vi "defaults.vi"(1 "Do this?":bool=TRUE, 2 "Input":i32[][](array[numeric]), 3 "Absolute start time (ms)":dbl format="%.3f") -> (0 "Output":i32[][](array[numeric])=[[0, 0, 0, 0], [0, 0, 0, 0], [0, 0, 0, 0], [0, 0, 0, 0], [0, 0, 0, 0], [0, 0, 0, 0], [0, 0, 0, 0], [0, 0, 0, 0], [0, 0, 0, 0], [0, 0, 0, 0], [0, 0, 0, 0], [0, 0, 0, 0], [0, 0, 0, 0], [0, 0, 0, 0], [0, 0, 0, 0], [0, 0, 0, 0], [0, 0, 0, 0], [0, 0, 0, 0], [0, 0, 0, 0], [0, 0, 0, 0], [0, 0, 0, 0], [0, 0, 0, 0], [0, 0, 0, 1], [0, 0, 0, 1], [0, 0, 0, 1], [0, 0, 0, 1], [0, 0, 0, 1], [0, 0, 0, 1], [0, 0, 0, 1], [0, 0, 0, 1], [0, 0, 0, 1], [0, 0, 0, 1], [0, 0, 0, 1], [0, 0, 1, 0], [0, 0, 2, 0], [0, 0, 3, 0], [0, 0, 4, 0], [0, 0, 5, 1], [0, 0, 6, 1], [0, 0, 7, 1], [0, 0, 8, 0], [0, 0, 9, 1], [0, 0, 10, 0], [0, 0, 11, 0], [0, 0, 12, 0], [0, 0, 13, 0], [0, 0, 14, 1], [0, 0, 15, 1], [0, 1, 0, 1], [0, 1, 1, 1], [0, 1, 2, 0], [0, 1, 3, 0], [0, 1, 4, 0], [0, 1, 5, 1], [0, 1, 6, 0], [0, 1, 7, 0], [0, 1, 8, 0], [0, 1, 9, 0], [0, 1, 10, 1], [0, 1, 11, 0], [0, 1, 12, 1], [0, 1, 13, 0], [0, 1, 14, 0], [0, 1, 15, 0]] caption="time(ms)        port            line               value")   [LabVIEW 2015]
uses:
  globals and logs/board parameters.vi
  globals and logs/modules globals.vi
panel:
  out "Defaults":bool[][](array[boolean])=[[FALSE, FALSE, FALSE, FALSE, FALSE, TRUE, TRUE, TRUE, FALSE, TRUE, FALSE, FALSE, FALSE, FALSE, TRUE, TRUE], [TRUE, TRUE, FALSE, FALSE, FALSE, TRUE, FALSE, FALSE, FALSE, FALSE, TRUE, FALSE, TRUE, FALSE, FALSE, FALSE], [FALSE, FALSE, FALSE, FALSE, FALSE, TRUE, TRUE, TRUE, FALSE, TRUE, FALSE, FALSE, FALSE, FALSE, TRUE, TRUE], [TRUE, TRUE, FALSE, FALSE, FALSE, TRUE, FALSE, FALSE, FALSE, FALSE, TRUE, FALSE, TRUE, FALSE, FALSE, FALSE]]
  out "Value":bool[](array[boolean])=[FALSE, FALSE, FALSE, FALSE, FALSE, TRUE, TRUE, TRUE, FALSE, TRUE, FALSE, FALSE, FALSE, FALSE, TRUE, TRUE, TRUE, TRUE, FALSE, FALSE, FALSE, TRUE, FALSE, FALSE, FALSE, FALSE, TRUE, FALSE, TRUE, FALSE, FALSE, FALSE, FALSE, FALSE, FALSE, FALSE, FALSE, TRUE, TRUE, TRUE, FALSE, TRUE, FALSE, FALSE, FALSE, FALSE, TRUE, TRUE, TRUE, TRUE, FALSE, FALSE, FALSE, TRUE, FALSE, FALSE, FALSE, FALSE, TRUE, FALSE, TRUE, FALSE, FALSE, FALSE]
  out "Line":i32[](array[numeric])=[0, 1, 2, 3, 4, 5, 6, 7, 8, 9, 10, 11, 12, 13, 14, 15, 0, 1, 2, 3, 4, 5, 6, 7, 8, 9, 10, 11, 12, 13, 14, 15]
  out "Port":i32[](array[numeric])=[0, 0, 0, 0, 0, 0, 0, 0, 0, 0, 0, 0, 0, 0, 0, 0, 1, 1, 1, 1, 1, 1, 1, 1, 1, 1, 1, 1, 1, 1, 1, 1]
  out "Time":dbl[](array[numeric]) format="%.3f"
  # "This subVI assembles a time,port,line,value array from the default values and the absolute start time.\nThis array is then added to the Input array.  If \"Do this?\" is False, then the Output array is just the Input array."
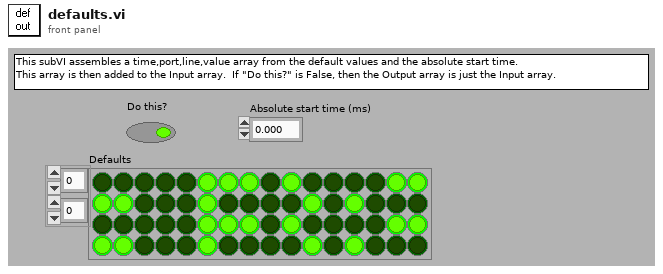
[diagram p1: front panel]
types:
  T1 = cluster{"Port":u32, "Line":u32, "Description":string, "Default":bool}[][]
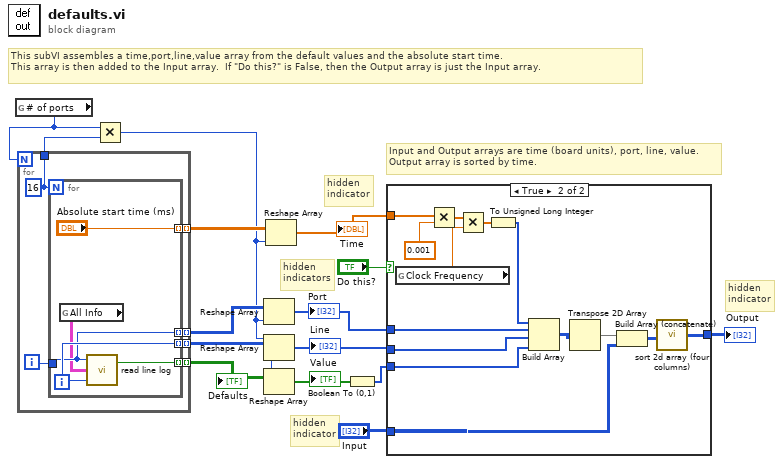
[diagram p0: block diagram]
diagram:
  # "hidden\nindicator"
  # "hidden\nindicator"
  # "hidden\nindicator"
  # "hidden\nindicators"
  # "This subVI assembles a time,port,line,value array from the default values and the absolute start time.\nThis array is then added to the Input array.  If \"Do this?\" is False, then the Output array is just the Input array."
  # "Input and Output arrays are time (board units), port, line, value.\nOutput array is sorted by time."
  n1 = global read "board parameters.vi" "# of ports"() -> (w1:u16)
  n2 = for {
    N: w1 -> [_]
    tunnel: [w20] -> w9 mode=indexing
    tunnel: [w19] -> w10 mode=indexing
    tunnel: [w17] -> w14 mode=indexing
    tunnel: [w18] -> w12 mode=indexing
    tunnel: [w16] -> w13
    i -> [w21]
    w16 = 16
    n3 = for {
      N: w16 -> [_]
      tunnel: [w23] -> w20 mode=indexing
      tunnel: w21 -> [w24]
      tunnel: [w25] -> w19 mode=indexing
      tunnel: [w24] -> w17 mode=indexing
      tunnel: ["Absolute start time (ms)"] -> w18 mode=indexing
      i -> [w25]
      n4 = global read "modules globals.vi" "All Info"() -> (w22:T1)
      n5 = call "read line log.vi"("Line"=w25, "All Info"=w22, "Port"=w24) -> ("Default  Value"=w23:bool)  [unwired: 1 out]
    }
  }
  "Defaults" <- w9
  n6 = Multiply(x=w1, y=w13) -> (x*y=w11:i32)
  n7 = Reshape Array(w14, w11) -> (w2:i32[])
  "Port" <- w2
  n8 = Reshape Array(w10, w11) -> (w5:i32[])
  "Line" <- w5
  n9 = Reshape Array(w9, w11) -> (w8:bool[])
  "Value" <- w8
  n10 = Reshape Array(w12, w11) -> (w7:dbl[])
  "Time" <- w7
  n11 = Boolean To (0,1)(Boolean=w8) -> (0, 1=w3:i16[])
  n12 = case shown="True" "Do this?" {
    tunnel: "Input" -> [w27 w28]
    tunnel: [w27 w41] -> w4
    tunnel: w7 -> [_ w36]
    tunnel: w5 -> [_ w33]
    tunnel: w3 -> [_ w34]
    tunnel: w2 -> [_ w32]
    frame False {
    }
    frame True {
      n13 = global read "board parameters.vi" "Clock Frequency"() -> (w38:dbl)
      n14 = Multiply(x=w36, y=0.001) -> (x*y=w39:dbl[])
      n15 = Multiply(x=w39, y=w38) -> (x*y=w37:dbl[])
      n16 = To Unsigned Long Integer(number=w37) -> (unsigned 32bit integer=w35:u32[])
      n17 = Build Array(w35, w32, w33, w34) -> (w31:u32[][])
      n18 = Transpose 2D Array(2D array=w31) -> (transposed array=w30:u32[][])
      n19 = Build Array (concatenate)(w30, w28) -> (w29:u32[][])
      n20 = call "sort 2d array (four columns).vi"("2D array to sort"=w29) -> ("Sorted array"=w41:i32[][])
    }
  }
  "Output" <- w4
